vi "-8441 CSV empty--error.vi"(8 "error in":errorcluster) -> (0 "error out":errorcluster)   [LabVIEW 2024, in "Named Fields Parser.lvclass"]
uses:
  Named Fields Parser.lvclass
  Named Fields Parser.lvclass/Named Fields Parser.ctl
  Common-LabVIEW-Helpers/Source/Error Helpers.lvlib
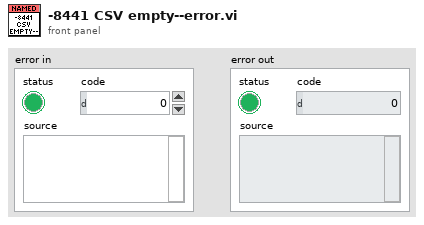
[diagram p1: front panel]
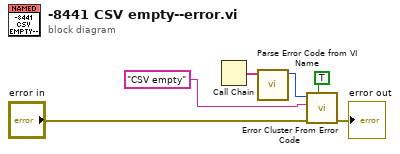
[diagram p0: block diagram]
diagram:
  n1 = Call Chain() -> (call chain=w3:string[])
  n2 = call "Parse Error Code from VI Name.vi"("Call Chain"=w3) -> ("Error Code"=w2:i32)  [unwired: 10 in]
  n3 = call <vilib>:"Error Cluster From Error Code.vi"("show call chain? (False)"=TRUE, "error in (no error)"="error in", "error message (\"\")"="CSV empty" ("source"), "error code (0)"=w2) -> ("error out"=→"error out":errorcluster)  [unwired: 5 in]
